vi "关键参数交互.vi"(9 "量程下拉列表":refnum<vi>, 10 "测量模式下拉列表":refnum<vi>, 11 "测量参数":refnum<vi>) -> ()   [LabVIEW 2016, in "斯坦道总氮.lvlib"]
panel:
  out "x != y?":T1
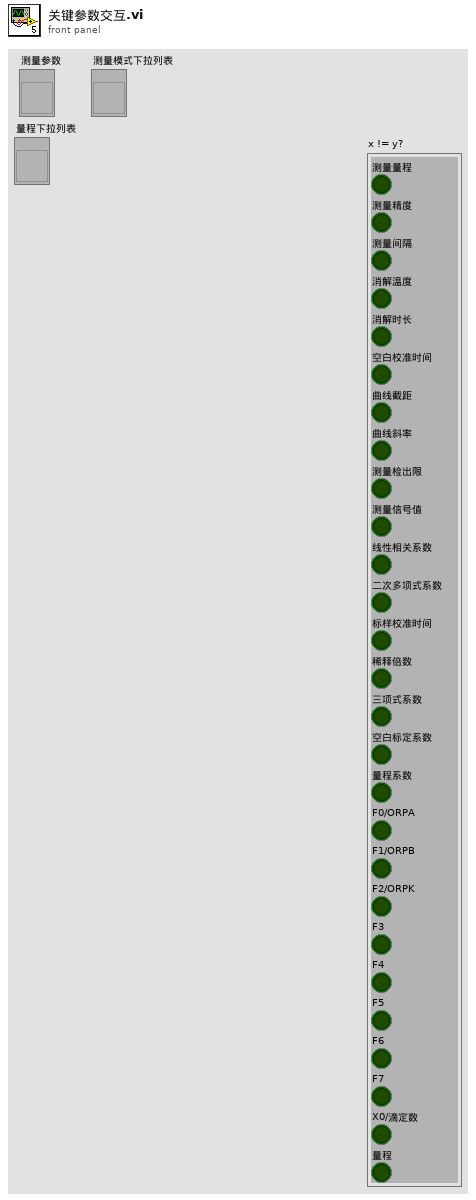
[diagram p1: front panel]
types:
  T1 = cluster{"测量量程":bool, "测量精度":bool, "测量间隔":bool, "消解温度":bool, "消解时长":bool, "空白校准时间":bool, "曲线截距":bool, "曲线斜率":bool, "测量检出限":bool, "测量信号值":bool, "线性相关系数":bool, "二次多项式系数":bool, "标样校准时间":bool, "稀释倍数":bool, "三项式系数":bool, "空白标定系数":bool, "量程系数":bool, "F0/ORPA":bool, "F1/ORPB":bool, "F2/ORPK":bool, "F3":bool, "F4":bool, "F5":bool, "F6":bool, "F7":bool, "X0/滴定数":bool, "量程":bool}
  T2 = cluster{"chose":string, "公式":cluster{"X^2":dbl, "X":dbl, "b":dbl}}
  T3 = cluster{"测量量程":dbl, "测量精度":dbl, "测量间隔":dbl, "消解温度":dbl, "消解时长":dbl, "空白校准时间":timestamp, "曲线截距":dbl, "曲线斜率":dbl, "测量检出限":dbl, "测量信号值":dbl, "线性相关系数":dbl, "二次多项式系数":dbl, "标样校准时间":timestamp, "稀释倍数":dbl, "三项式系数":dbl, "空白标定系数":dbl, "量程系数":dbl, "F0/ORPA":dbl, "F1/ORPB":dbl, "F2/ORPK":dbl, "F3":dbl, "F4":dbl, "F5":dbl, "F6":dbl, "F7":dbl, "X0/滴定数":dbl, "量程":dbl}
  T4 = cluster{"时间标识":timestamp, "设备":string, "日志信息":string, "流程参数":string}
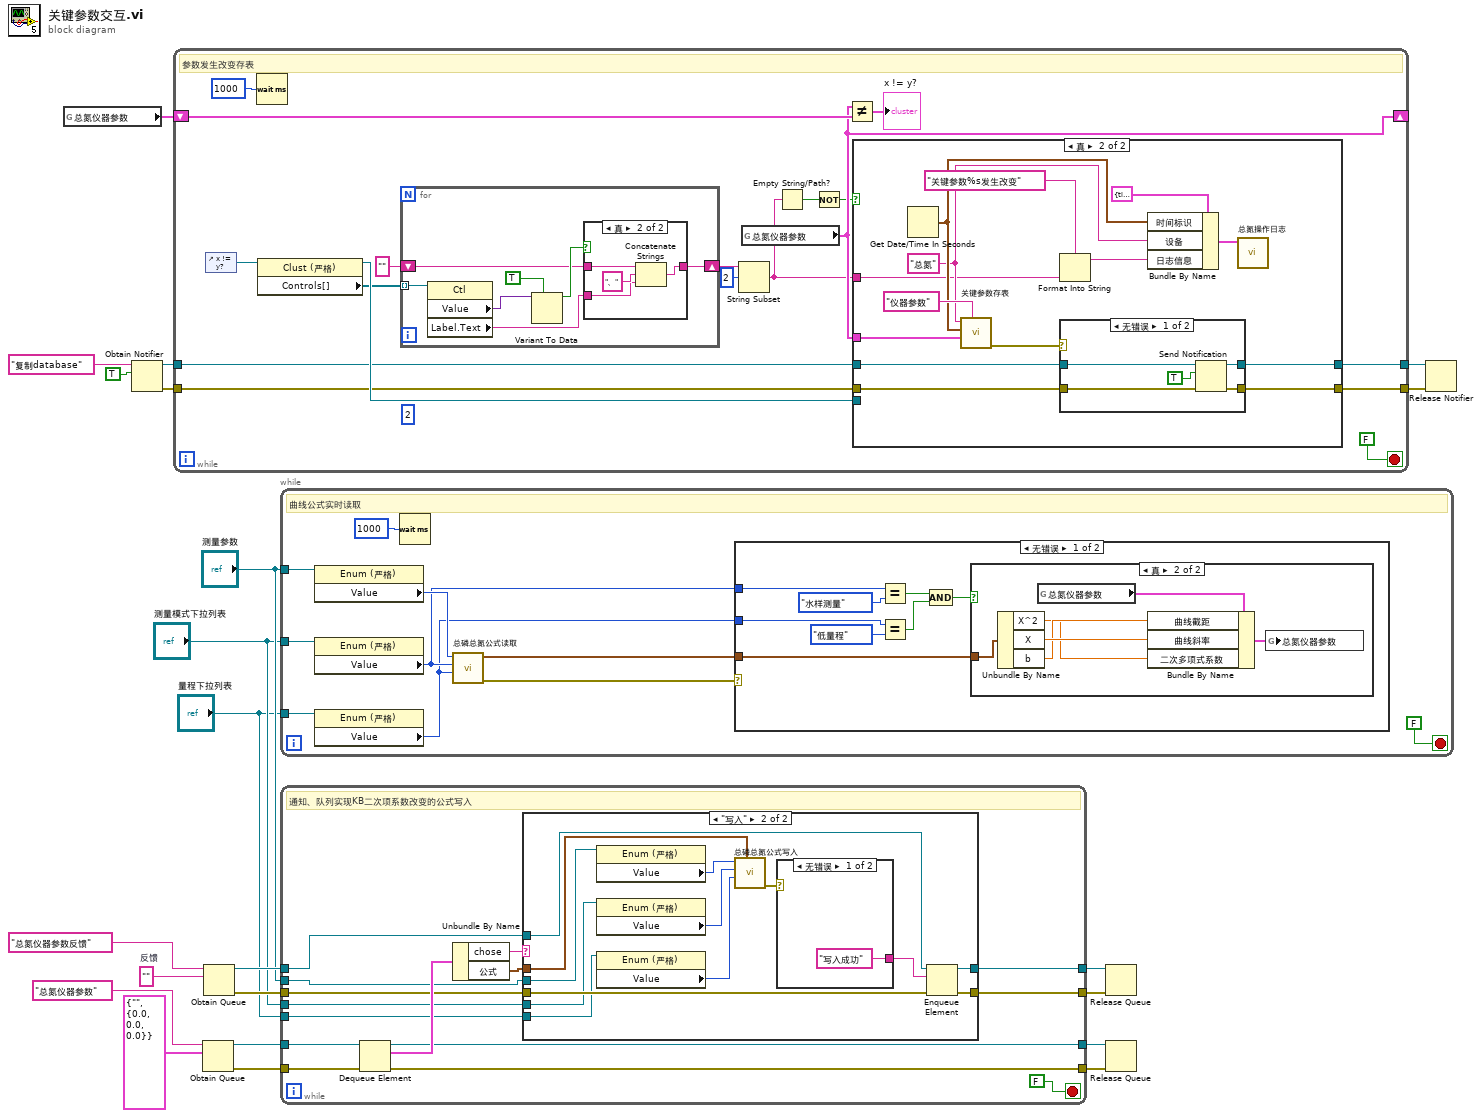
[diagram p0: block diagram]
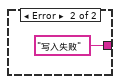
[diagram p5: hidden frame]
diagram:
  w13 = ""  # 反馈
  n1 = global read "总氮断电保存全局变量.vi" "总氮仪器参数"() -> (w22:T3)
  n2 = Obtain Notifier(name (unnamed)="复制database" ("名称（未命名）"), notification data type=TRUE) -> (notifier out=w7:refnum<notifier>, error out=w6:errorcluster)  [unwired: 2 in, 1 out]
  n3 = while {
    shift-right: [w35] -> _
    shift-left: w22 -> [w38]
    tunnel: w7 -> [w33]
    tunnel: w6 -> [w32]
    tunnel: [w31] -> w5
    tunnel: [w30] -> w4
    stop <- FALSE stop-if-true
    (unwired) 2 ("偏移量(0)")
    # "参数发生改变存表"
    n4 = control-ref of="x != y?"() -> (w36:refnum<vi>)
    n5 = Wait (ms)(milliseconds to wait=u32 1000 ("等待时间（毫秒）")) -> ()  [unwired: 1 out]
    n6 = property class="Clust (严格)"(reference=w36) -> (reference out=w34:refnum<vi>, "Controls[]"=w26:refnum<vi>[])  [unwired: 1 in, 1 out]
    n7 = for {
      tunnel: w26 -> [w47] mode=indexing
      shift-right: [w41] -> w28
      shift-left: "" -> [w43]
      n8 = property class="Ctl"(reference=w47) -> ("Value"=w45:variant, "Label.Text"=w42:string)  [unwired: 1 in, 2 out]
      n9 = Variant To Data(type=TRUE, Variant=w45) -> (data=w44:bool)  [unwired: 1 in, 1 out]
      n10 = case shown="真" w44 {
        tunnel: w43 -> [w48 w52]
        tunnel: w42 -> [_ w49]
        tunnel: [w48 w51] -> w41
        frame False {
        }
        frame True {
          n11 = Concatenate Strings(w52, "、", w49) -> (w51:string)
        }
      }
    }
    n12 = String Subset(string=w28, offset (0)=2 ("偏移量(0)")) -> (substring=w25:string)  [unwired: 1 in]
    n13 = global read "总氮断电保存全局变量.vi" "总氮仪器参数"() -> (w35:T3)
    n14 = Empty String/Path?(string/path=w25) -> (empty?=w29:bool)
    n15 = Not(x=w29) -> (.not. x?=w24:bool)
    n16 = Not Equal?(x=w35, y=w38) -> (x != y?=→"x != y?":T1)
    n17 = case shown="真" w24 {
      tunnel: w35 -> [_ w67]
      tunnel: w25 -> [_ w61]
      tunnel: w34 -> [_ _]
      tunnel: w33 -> [w53 w58]
      tunnel: w32 -> [w54 w57]
      tunnel: [w53 w56] -> w31
      tunnel: [w54 w55] -> w30
      frame False {
      }
      frame True {
        w63 = "总氮" ("仪器名称")
        n18 = Get Date/Time In Seconds() -> (seconds since 1Jan1904=w64:timestamp)
        n19 = call "关键参数存表.vi"("table"="仪器参数", "仪器参数"=w67, "datatime"=w64, "仪器名称"=w63) -> ("error out"=w59:errorcluster)  [unwired: 7 in]
        n20 = Format Into String(format string="关键参数%s发生改变" ("格式字符串"), w61) -> (resulting string=w60:string)  [unwired: 2 in, 1 out]
        n21 = case shown="无错误" w59 {
          tunnel: w58 -> [w73 w75]
          tunnel: w57 -> [w72 w74]
          tunnel: [w70 w75] -> w56
          tunnel: [w69 w74] -> w55
          frame No Error {
            n22 = Send Notification(notification=TRUE ("通知"), notifier=w73, error in (no error)=w72) -> (notifier out=w70:refnum<notifier>, error out=w69:errorcluster)
          }
          frame Error {
          }
        }
        n23 = Bundle By Name(cluster=T4 {"时间标识"=timestamp(0 s since 1904-01-01), "设备"="", "日志信息"="", "流程参数"=""} ("data in"), "时间标识"=w64, "设备"=w63, "日志信息"=w60) -> (w65:T4)
        n24 = call "总氮操作日志.vi"("data in"=w65) -> ()  [unwired: 11 in]
      }
    }
  }
  n25 = Obtain Queue(name (unnamed)="总氮仪器参数" ("名称（未命名）"), element data type=T2 {"chose"="", "公式"={"X^2"=0.0, "X"=0.0, "b"=0.0}}) -> (queue out=w21:refnum<queue>, error out=w20:errorcluster)  [unwired: 3 in, 1 out]
  n26 = Obtain Queue(name (unnamed)="总氮仪器参数反馈" ("名称（未命名）"), element data type=w13) -> (queue out=w14:refnum<queue>, error out=w12:errorcluster)  [unwired: 3 in, 1 out]
  n27 = while {
    tunnel: "测量参数" -> [w83]
    tunnel: "测量模式下拉列表" -> [w82]
    tunnel: "量程下拉列表" -> [w81]
    stop <- FALSE stop-if-true
    # "曲线公式实时读取"
    n28 = property class="Enum (严格)"(reference=w83) -> ("Value"=w80:enum16{"总磷", "总氮"})  [unwired: 1 in, 2 out]
    n29 = property class="Enum (严格)"(reference=w82) -> ("Value"=w79:enum16{"水样测量", "零点核查", "跨度核查", "标样核查", "加标回收"})  [unwired: 1 in, 2 out]
    n30 = property class="Enum (严格)"(reference=w81) -> ("Value"=w78:enum16{"低量程", "高量程"})  [unwired: 1 in, 2 out]
    n31 = Wait (ms)(milliseconds to wait=u32 1000 ("等待时间（毫秒）")) -> ()  [unwired: 1 out]
    n32 = call "总磷总氮公式读取.vi"("量程"=w78, "测量模式"=w79, "测量参数"=w80) -> ("error out"=w77:errorcluster, "公式"=w76:cluster{"X^2":dbl, "X":dbl, "b":dbl})  [unwired: 7 in]
    n33 = case shown="无错误" w77 {
      tunnel: w79 -> [w93 _]
      tunnel: w76 -> [w87 _]
      tunnel: w78 -> [w86 _]
      frame No Error {
        n34 = Equal?(x=w93, y=enum16{"水样测量", "零点核查", "跨度核查", "标样核查", "加标回收"}."水样测量") -> (x = y?=w90:bool)
        n35 = Equal?(x=w86, y=enum16{"低量程", "高量程"}."低量程") -> (x = y?=w89:bool)
        n36 = Compound Arithmetic op=AND ("复合运算")(w90, w89) -> (w88:bool)
        n37 = case shown="真" w88 {
          tunnel: w87 -> [_ w99]
          frame False {
          }
          frame True {
            n38 = Unbundle By Name(w99) -> ("X^2"=w96:dbl, "X"=w98:dbl, "b"=w97:dbl)
            n39 = global read "总氮断电保存全局变量.vi" "总氮仪器参数"() -> (w95:T3)
            n40 = Bundle By Name(cluster=w95, "曲线截距"=w97, "曲线斜率"=w98, "二次多项式系数"=w96) -> (w94:T3)
            n41 = global write "总氮断电保存全局变量.vi" "总氮仪器参数"(w94) -> ()
          }
        }
      }
      frame Error {
      }
    }
  }
  n42 = while {
    tunnel: w21 -> [w113]
    tunnel: w20 -> [w112]
    tunnel: [w108] -> w17
    tunnel: [w107] -> w16
    tunnel: w14 -> [w106]
    tunnel: w12 -> [w105]
    tunnel: [w104] -> w11
    tunnel: [w103] -> w10
    tunnel: "测量参数" -> [w102]
    tunnel: "测量模式下拉列表" -> [w101]
    tunnel: "量程下拉列表" -> [w100]
    stop <- FALSE stop-if-true
    # "通知、队列实现KB二次项系数改变的公式写入"
    n43 = Dequeue Element(queue=w113, error in (no error)=w112) -> (queue out=w108:refnum<queue>, element=w111:T2, error out=w107:errorcluster)  [unwired: 1 in, 1 out]
    n44 = Unbundle By Name(w111) -> ("chose"=w110:string, "公式"=w109:cluster{"X^2":dbl, "X":dbl, "b":dbl})
    n45 = case shown="\"写入\"" w110 {
      tunnel: w109 -> [_ w126]
      tunnel: w106 -> [w116 w125]
      tunnel: w105 -> [w115 w123]
      tunnel: [w116 w122] -> w104
      tunnel: [w115 w121] -> w103
      tunnel: w102 -> [_ w119]
      tunnel: w101 -> [_ w118]
      tunnel: w100 -> [_ w117]
      frame "假", Default {
      }
      frame "写入" {
        n46 = property class="Enum (严格)"(reference=w119) -> ("Value"=w120:enum16{"总磷", "总氮"})  [unwired: 1 in, 2 out]
        n47 = property class="Enum (严格)"(reference=w118) -> ("Value"=w128:enum16{"水样测量", "零点核查", "跨度核查", "标样核查", "加标回收"})  [unwired: 1 in, 2 out]
        n48 = property class="Enum (严格)"(reference=w117) -> ("Value"=w129:enum16{"低量程", "高量程"})  [unwired: 1 in, 2 out]
        n49 = call "总磷总氮公式写入.vi"("公式"=w126, "量程"=w129, "测量模式"=w128, "测量参数"=w120) -> ("error out"=w127:errorcluster)  [unwired: 7 in]
        n50 = case shown="无错误" w127 {
          tunnel: ["写入成功" ("消息") "写入失败" ("消息")] -> w124
          frame No Error {
          }
          frame Error {
          }
        }
        n51 = Enqueue Element(queue=w125, element=w124, error in (no error)=w123) -> (queue out=w122:refnum<queue>, error out=w121:errorcluster)  [unwired: 1 in, 1 out]
      }
    }
  }
  n52 = Release Queue(queue=w11, error in (no error)=w10) -> ()  [unwired: 1 in, 3 out]
  n53 = Release Queue(queue=w17, error in (no error)=w16) -> ()  [unwired: 1 in, 3 out]
  n54 = Release Notifier(notifier=w5, error in (no error)=w4) -> ()  [unwired: 1 in, 3 out]
